vi "Can Add Timing Channels.vi"(8 "error in (no error)":errorcluster, 9 "Menu heirarchy in":string[](array[string]), 11 "Node Ptr":T2 format="%.0x") -> (0 "error out":errorcluster, 1 "Menu heirarchy out":string[](array[string]), 3 "Action":T1)   [LabVIEW 2024, in "AIM ARINC 429 System Explorer.lvlib"]
uses:
  AIM ARINC 429 System Explorer.lvlib
  Includes/AIM ARINC 429 System Explorer.lvlibp/1abvi3w/vi.lib/NI VeriStand/Custom Device API/Custom Device Item Ref.ctl
  Includes/AIM ARINC 429 System Explorer.lvlibp/1abvi3w/vi.lib/NI VeriStand/Custom Device API/Custom Device RTM Dependency.ctl
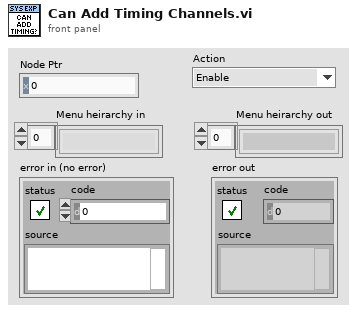
[diagram p1: front panel]
types:
  T1 = typedef "AIM ARINC 429 System Explorer.lvlibp/Custom Device API.lvlib/Custom Device RTM Dependency.ctl" = enum16{"Enable", "Disable", "Hide"}
  T2 = typedef "AIM ARINC 429 System Explorer.lvlibp/Custom Device API.lvlib/Custom Device Item Ref.ctl" = u64
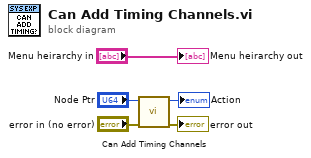
[diagram p0: block diagram]
diagram:
  n1 = call "Can Add Timing Channels.vi"("error in"="error in (no error)", "Node Ptr"="Node Ptr") -> ("error out"=→"error out":errorcluster, "Action"=→"Action":T1)  [unwired: 8 in]
  "Menu heirarchy out" <- "Menu heirarchy in"
